vi "Surrey.vi"(8 "Target Speed":dbl caption="RPM" format="%.1f", 11 "Fan on Button":bool) -> ()   [LabVIEW 2010]
panel:
  in  "Stop Road Drive":bool
  in  "PitotZero button":bool
  in  "Stop HS Logging":bool
  in  "Start HS Logging":bool
  out "SmAD Data String":string
  in  "SmAD":bool caption="V&H offsets"
  out "Fan Running":bool
  out "Yaw Ready":bool caption="Ready"
  in  "Start Road Drive":bool
  out "P (mbar)":dbl caption="Current Setting" format="%.2f"
  in  "Set \"X\"Offset (mm)":dbl caption="0.000000" format="%.1f"
  in  "Quit":bool
  out "Road Ready":bool
  out "Road Fault":bool
  in  "Road Stop Button":bool
  out "Road Speed":dbl caption="m/s"
  in  "road speed selection":enum32{"road manual", "road sync to wind"}(radio)
  in  "Road target speed":dbl caption="Target  Speed" format="%.1f"
  in  "Road set speed  Button":bool caption="Set Speed"
  out "E-Stop Active":bool
  in  "Fan Stop button":bool
  in  "Fan radio buttons":T1(radio)
  out "Yaw Complete":bool caption="Complete"
  out "Yaw Limits":bool caption="Limits"
  out "Yaw Moving":bool caption="Moving"
  in  "yaw stop button":bool
  in  "Yaw GO Button":bool
  in  "Required Yaw":dbl format="%.2f"
  out "Yaw position":dbl(knob) caption="Degrees" scale=-5.0..5.0 scale format="%#_6f"
  in  "Update Balance Offsets":bool caption="V&H offsets"
  in  "Set \"Z\"Offset (mm)":dbl caption="0.000000" format="%.1f"
  in  "Data Net Button":bool
  in  "data ABS button":bool
  in  "SigConSetup":bool
  in  "Numeric Zero(All Axis) button":bool caption="Numeric Zero(All Axis)"
  in  "Boro Update":bool
  out "T (deg)":dbl caption="C"
  in  "P (mbar)":dbl caption="etting" format="%.2f"
  in  "E_STOP ALL":bool
  out "Fan Ready":bool
  out "Fan Speed":dbl caption="RPM"
  out "Wind Speed":dbl caption="m/s"
  in  "fan Set Speed":bool
  out "Roll gauge":dbl(slide) caption="100%             0                -100%" scale=-100.0..100.0
  out "Roll":dbl caption="N.m" format="%#.2f"
  out "Yaw gauge":dbl(slide) caption="100%             0                -100%" scale=-100.0..100.0
  out "Yaw":dbl caption="N.m" format="%#.2f"
  out "Side-force gauge":dbl(slide) caption="100%             0                -100%" scale=-100.0..100.0
  out "Side-Force":dbl caption="N" format="%#.2f"
  out "Drag Gauge":dbl(slide) caption="100%             0                -100%" scale=-100.0..100.0
  out "Drag":dbl caption="N" format="%#.2f"
  out "Pitch gauge":dbl(slide) caption="100%             0                -100%" scale=-100.0..100.0
  out "Pitch":dbl caption="N.m" format="%#.2f"
  out "Lift gauge":dbl(slide) caption="100%             0                -100%" scale=-100.0..100.0
  out "Lift":dbl caption="N" format="%#.2f"
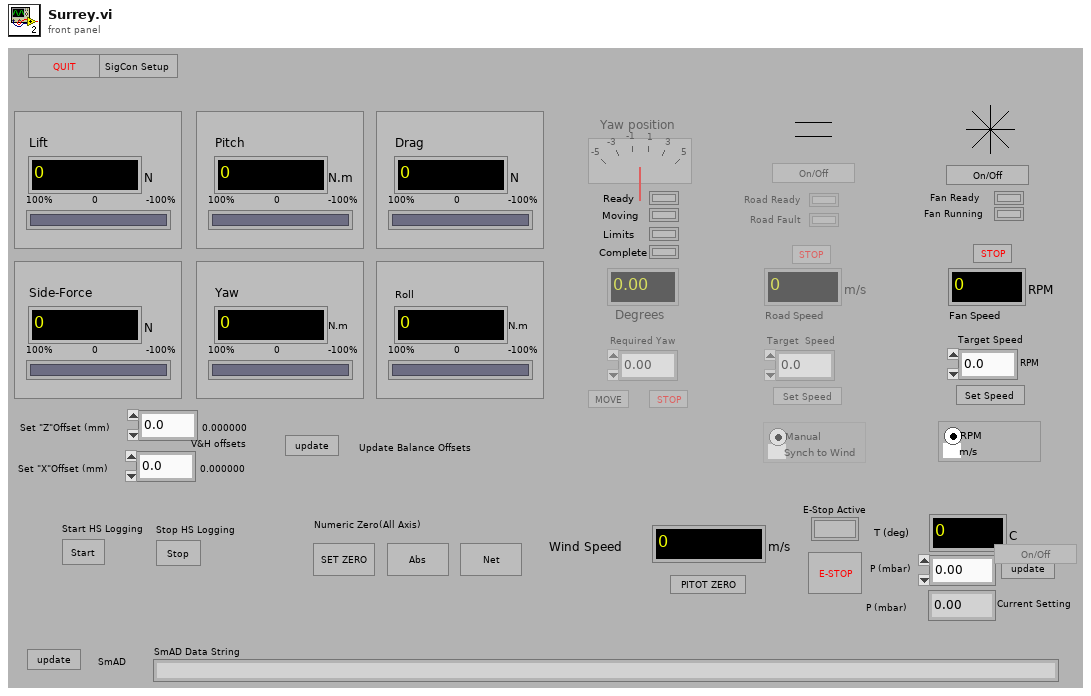
[diagram p1: front panel]
types:
  T1 = enum32{"Fan Control Selection  in RPM", "Fan speed option m/s"}
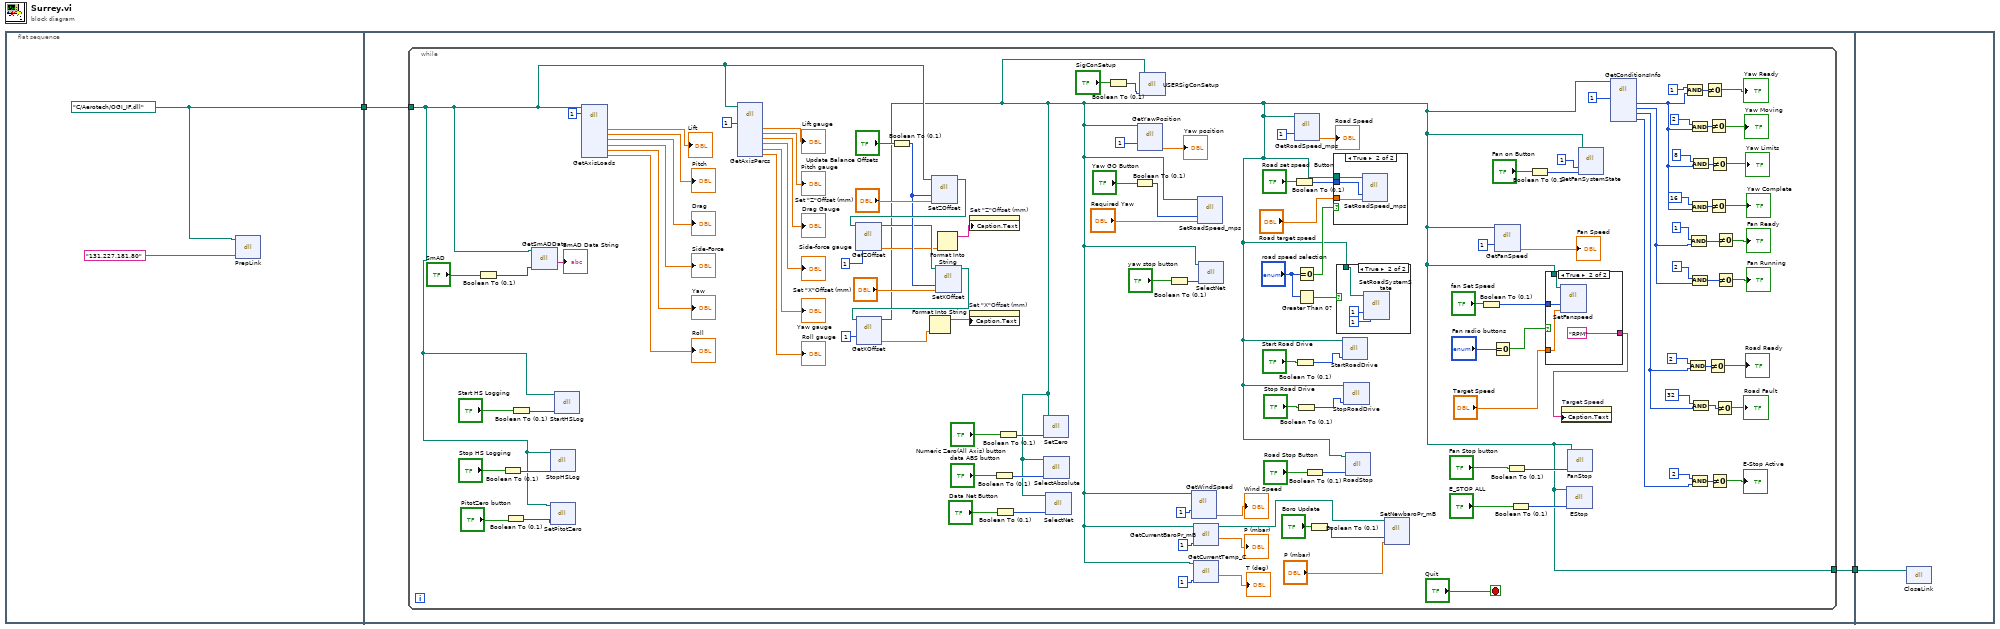
[diagram p0: block diagram]
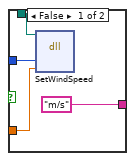
[diagram p4: hidden frame]
diagram:
  n1 = flat-sequence {
    tunnel: [w4] -> w2
    tunnel: w2 -> [w6]
    tunnel: [w5] -> w1
    tunnel: w1 -> [w146]
    frame #0 {
      w4 = path "C:/Aerotech/OGI_IF.dll" ("path in")
      n2 = dll-call lib="C:/Aerotech/Drivers/OGI_IF.dll" fn="PrepLink"(path in=w4, "IPAddress"="131.227.181.80") -> ()  [unwired: 2 in, 4 out]
    }
    frame #1 {
      n3 = while {
        tunnel: w6 -> [w11]
        tunnel: [w7] -> w5
        stop <- "Quit" stop-if-true
        n4 = Boolean To (0,1)(Boolean="SmAD") -> (0, 1=w18:i16)
        n5 = Boolean To (0,1)(Boolean="Stop HS Logging") -> (0, 1=w14:i16)
        n6 = Boolean To (0,1)(Boolean="PitotZero button") -> (0, 1=w12:i16)
        n7 = Boolean To (0,1)(Boolean="Start HS Logging") -> (0, 1=w17:i16)
        n8 = dll-call lib="C:/Aerotech/Drivers/OGI_IF.dll" fn="GetSmADData"(path in=w11, "Enable"=w18) -> ("SmAD Data String"=→"SmAD Data String":string)  [unwired: 2 in, 3 out]
        n9 = dll-call lib="C:/Aerotech/Drivers/OGI_IF.dll" fn="StopHSLog"(path in=w11, "Enable"=w14) -> ()  [unwired: 2 in, 4 out]
        n10 = dll-call lib="C:/Aerotech/Drivers/OGI_IF.dll" fn="SetPitotZero"(path in=w11, "Enable"=w12) -> ()  [unwired: 2 in, 4 out]
        n11 = dll-call lib="C:/Aerotech/Drivers/OGI_IF.dll" fn="StartHSLog"(path in=w11, "Enable"=w17) -> ()  [unwired: 2 in, 4 out]
        n12 = dll-call lib="C:/Aerotech/Drivers/OGI_IF.dll" fn="GetAxisLoads"(path in=w11, "Enable"=1) -> ("Lift"=→"Lift":dbl, "Pitch"=→"Pitch":dbl, "Drag"=→"Drag":dbl, "side"=→"Side-Force":dbl, "Yaw"=→"Yaw":dbl, "Roll"=→"Roll":dbl)  [unwired: 3 in, 9 out]
        n13 = dll-call lib="C:/Aerotech/Drivers/OGI_IF.dll" fn="GetAxisPercs"(path in=w11, "Enable"=1) -> ("Lift"=→"Lift gauge":dbl, "Pitch"=→"Pitch gauge":dbl, "Drag"=→"Drag Gauge":dbl, "side"=→"Side-force gauge":dbl, "Yaw"=→"Yaw gauge":dbl, "Roll"=→"Roll gauge":dbl)  [unwired: 3 in, 9 out]
        n14 = Boolean To (0,1)(Boolean="Update Balance Offsets") -> (0, 1=w115:i16)
        n15 = dll-call lib="C:/Aerotech/Drivers/OGI_IF.dll" fn="SetZOffset"(path in=w11, "Enable"=w115, "SetZoffset"="Set \"Z\"Offset (mm)") -> (path out=w116:path)  [unwired: 3 in, 3 out]
        n16 = dll-call lib="C:/Aerotech/Drivers/OGI_IF.dll" fn="GetZOffset"(path in=w116, "Enable"=1) -> (path out=w112:path, "ZOffset"=w28:dbl)  [unwired: 3 in, 3 out]
        n17 = dll-call lib="C:/Aerotech/Drivers/OGI_IF.dll" fn="SetXOffset"(path in=w112, "Enable"=w115, "SetXOffset"="Set \"X\"Offset (mm)") -> (path out=w111:path)  [unwired: 3 in, 3 out]
        n18 = dll-call lib="C:/Aerotech/Drivers/OGI_IF.dll" fn="GetXOffset"(path in=w111, "Enable"=1) -> (path out=w7:path, "XOffset"=w26:dbl)  [unwired: 3 in, 3 out]
        n19 = Format Into String(w26) -> (resulting string=w114:string)  [unwired: 3 in, 1 out]
        n20 = Format Into String(w28) -> (resulting string=w27:string)  [unwired: 3 in, 1 out]
        n21 = property on="Set \"X\"Offset (mm)" class="DigNum (strict)"("Caption.Text"=w114) -> ()  [unwired: 2 in, 2 out]
        n22 = property on="Set \"Z\"Offset (mm)" class="DigNum (strict)"("Caption.Text"=w27) -> ()  [unwired: 2 in, 2 out]
        n23 = Boolean To (0,1)(Boolean="data ABS button") -> (0, 1=w103:i16)
        n24 = Boolean To (0,1)(Boolean="Data Net Button") -> (0, 1=w106:i16)
        n25 = Boolean To (0,1)(Boolean="Numeric Zero(All Axis) button") -> (0, 1=w109:i16)
        n26 = dll-call lib="C:/Aerotech/Drivers/OGI_IF.dll" fn="SetZero"(path in=w7, "Enable"=w109) -> ()  [unwired: 2 in, 4 out]
        n27 = dll-call lib="C:/Aerotech/Drivers/OGI_IF.dll" fn="SelectAbsolute"(path in=w7, "Enable"=w103) -> ()  [unwired: 2 in, 4 out]
        n28 = dll-call lib="C:/Aerotech/Drivers/OGI_IF.dll" fn="SelectNet"(path in=w7, "Enable"=w106) -> ()  [unwired: 2 in, 4 out]
        n29 = Boolean To (0,1)(Boolean="SigConSetup") -> (0, 1=w92:i16)
        n30 = Boolean To (0,1)(Boolean="Yaw GO Button") -> (0, 1=w30:i16)
        n31 = dll-call lib="C:/Aerotech/Drivers/OGI_IF.dll" fn="GetYawPosition"(path in=w7, "Enable"=1) -> ("YawPosDeg"=→"Yaw position":dbl)  [unwired: 3 in, 4 out]
        n32 = dll-call lib="C:/Aerotech/Drivers/OGI_IF.dll" fn="USERSigConSetup"(path in=w7, "Enable"=w92) -> ()  [unwired: 2 in, 4 out]
        n33 = Boolean To (0,1)(Boolean="yaw stop button") -> (0, 1=w68:i16)
        n34 = dll-call lib="C:/Aerotech/Drivers/OGI_IF.dll" fn="GetWindSpeed"(path in=w7, "Enable"=1) -> ("Windspeed_M/s"=→"Wind Speed":dbl)  [unwired: 3 in, 4 out]
        n35 = dll-call lib="C:/Aerotech/Drivers/OGI_IF.dll" fn="GetCurrentBaroPr_mB"(path in=w7, "Enable"=1) -> (path out=w23:path, "mbar"=→"P (mbar)":dbl)  [unwired: 3 in, 1 out]
        n36 = dll-call lib="C:/Aerotech/Drivers/OGI_IF.dll" fn="GetCurrentTemp_C"(path in=w7, "Enable"=1) -> ("Deg_C"=→"T (deg)":dbl)  [unwired: 3 in, 2 out]
        n37 = dll-call lib="C:/Program Files/EnFlo Software/OGI_IF.dll" fn="SetRoadSpeed_mps"(path in=w7, "Enable"=w30, "NewRoadSpeed"="Required Yaw") -> ()  [unwired: 2 in, 5 out]
        n38 = dll-call lib="C:/Aerotech/Drivers/OGI_IF.dll" fn="SelectNet"(path in=w7, "Enable"=w68) -> ()  [unwired: 2 in, 4 out]
        n39 = dll-call lib="C:/Aerotech/Drivers/OGI_IF.dll" fn="GetRoadSpeed_mps"(path in=w7, "Enable"=1) -> ("RoadSpeedm/s"=→"Road Speed":dbl)  [unwired: 3 in, 4 out]
        n40 = Boolean To (0,1)(Boolean="Road set speed  Button") -> (0, 1=w78:i16)
        n41 = Boolean To (0,1)(Boolean="Start Road Drive") -> (0, 1=w10:i16)
        n42 = Equal To 0?(x="road speed selection") -> (x = 0?=w80:bool)
        n43 = Boolean To (0,1)(Boolean="Stop Road Drive") -> (0, 1=w8:i16)
        n44 = Greater Than 0?(x="road speed selection") -> (x > 0?=w75:bool)
        n45 = Boolean To (0,1)(Boolean="Road Stop Button") -> (0, 1=w72:i16)
        n46 = Boolean To (0,1)(Boolean="Boro Update") -> (0, 1=w22:i16)
        n47 = case shown="True" w80 {
          tunnel: w7 -> [_ w137]
          tunnel: w78 -> [_ w136]
          tunnel: "Road target speed" -> [_ w135]
          frame False {
          }
          frame True {
            n48 = dll-call lib="C:/Aerotech/OGI_IF.dll" fn="SetRoadSpeed_mps"(path in=w137, "Enable"=w136, "NewRoadSpeed"=w135) -> ()  [unwired: 3 in, 4 out]
          }
        }
        n49 = case shown="True" w75 {
          tunnel: w7 -> [_ w132]
          frame False {
          }
          frame True {
            n50 = dll-call lib="C:/Aerotech/Drivers/OGI_IF.dll" fn="SetRoadSystemState"(path in=w132, "Enable"=1, "RoadSyncToWind"=1) -> ()  [unwired: 4 in, 3 out]
          }
        }
        n51 = dll-call lib="C:/Aerotech/OGI_IF.dll" fn="StartRoadDrive"(path in=w7, "Enable"=w10) -> ()  [unwired: 3 in, 3 out]
        n52 = dll-call lib="C:/Aerotech/OGI_IF.dll" fn="StopRoadDrive"(path in=w7, "Enable"=w8) -> ()  [unwired: 3 in, 3 out]
        n53 = dll-call lib="C:/Aerotech/Drivers/OGI_IF.dll" fn="RoadStop"(path in=w7, "Enable"=w72) -> ()  [unwired: 2 in, 4 out]
        n54 = dll-call lib="C:/Aerotech/Drivers/OGI_IF.dll" fn="SetNewbaroPr_mB"(path in=w23, "Enable"=w22, "NewPressure"="P (mbar)") -> ()  [unwired: 3 in, 4 out]
        n55 = Boolean To (0,1)(Boolean="fan Set Speed") -> (0, 1=w32:i16)
        n56 = Equal To 0?(x="Fan radio buttons") -> (x = 0?=w96:bool)
        n57 = dll-call lib="C:/Aerotech/Drivers/OGI_IF.dll" fn="GetFanSpeed"(path in=w7, "Enable"=1) -> ("FanSpeedinRPM"=→"Fan Speed":dbl)  [unwired: 3 in, 4 out]
        n58 = Boolean To (0,1)(Boolean="Fan Stop button") -> (0, 1=w100:i16)
        n59 = Boolean To (0,1)(Boolean="E_STOP ALL") -> (0, 1=w84:i16)
        n60 = Boolean To (0,1)(Boolean="Fan on Button") -> (0, 1=w66:i16)
        n61 = case shown="True" w96 {
          tunnel: w7 -> [w141 w145]
          tunnel: w32 -> [w138 w144]
          tunnel: "Target Speed" -> [w140 w143]
          tunnel: ["m/s" "RPM"] -> w31
          frame False {
            n62 = dll-call lib="C:/Aerotech/Drivers/OGI_IF.dll" fn="SetWindSpeed"(path in=w141, "Enable"=w138, "NewWindSpeed"=w140) -> ()  [unwired: 3 in, 4 out]
          }
          frame True {
            n63 = dll-call lib="C:/Aerotech/Drivers/ATE_Surrey_WTCS.dll" fn="SetFanspeed"(path in=w145, "Enable"=w144, "NewFanSpeed"=w143) -> ()  [unwired: 3 in, 4 out]
          }
        }
        n64 = property on="Target Speed" class="DigNum (strict)"("Caption.Text"=w31) -> ()  [unwired: 2 in, 2 out]
        n65 = dll-call lib="C:/Aerotech/Drivers/OGI_IF.dll" fn="EStop"(path in=w7, "Enable"=w84) -> ()  [unwired: 2 in, 4 out]
        n66 = dll-call lib="C:/Aerotech/Drivers/OGI_IF.dll" fn="FanStop"(path in=w7, "Enable"=w100) -> ()  [unwired: 2 in, 4 out]
        n67 = dll-call lib="C:/Aerotech/Drivers/OGI_IF.dll" fn="SetFanSystemState"(path in=w7, "Enable"=1, "Fan ONOFF"=w66) -> ()  [unwired: 3 in, 4 out]
        n68 = dll-call lib="C:/Aerotech/Drivers/OGI_IF.dll" fn="GetConditionsInfo"(path in=w7, "Enable"=1) -> ("YawControl"=w45:i32, "FanControl"=w33:i32, "RoadControl"=w44:i32, "Globals"=w40:i32)  [unwired: 3 in, 7 out]
        n69 = Compound Arithmetic op=AND(1 ("value"), w45) -> (w65:i32)
        n70 = Compound Arithmetic op=AND(2 ("value"), w44) -> (w49:i32)
        n71 = Compound Arithmetic op=AND(1 ("value"), w33) -> (w53:i32)
        n72 = Compound Arithmetic op=AND(2 ("value"), w45) -> (w62:i32)
        n73 = Compound Arithmetic op=AND(16 ("value"), w45) -> (w60:i32)
        n74 = Compound Arithmetic op=AND(2 ("value"), w33) -> (w34:i32)
        n75 = Compound Arithmetic op=AND(2 ("value"), w40) -> (w43:i32)
        n76 = Compound Arithmetic op=AND(8 ("value"), w45) -> (w61:i32)
        n77 = Compound Arithmetic op=AND(32 ("value"), w44) -> (w48:i32)
        n78 = Not Equal To 0?(x=w65) -> (x != 0?=→"Yaw Ready":bool)
        n79 = Not Equal To 0?(x=w49) -> (x != 0?=→"Road Ready":bool)
        n80 = Not Equal To 0?(x=w62) -> (x != 0?=→"Yaw Moving":bool)
        n81 = Not Equal To 0?(x=w60) -> (x != 0?=→"Yaw Complete":bool)
        n82 = Not Equal To 0?(x=w61) -> (x != 0?=→"Yaw Limits":bool)
        n83 = Not Equal To 0?(x=w43) -> (x != 0?=→"E-Stop Active":bool)
        n84 = Not Equal To 0?(x=w48) -> (x != 0?=→"Road Fault":bool)
        n85 = Not Equal To 0?(x=w53) -> (x != 0?=→"Fan Ready":bool)
        n86 = Not Equal To 0?(x=w34) -> (x != 0?=→"Fan Running":bool)
      }
    }
    frame #2 {
      n87 = dll-call lib="C:/Aerotech/Drivers/OGI_IF.dll" fn="CloseLink"(path in=w146) -> ()  [unwired: 2 in, 3 out]
    }
  }
